vi "Inverter Test.vi"() -> ()   [LabVIEW 2016]
uses:
  <vilib>/TagLibrary/Create Tag (Int).vi
  <vilib>/TagLibrary/Write (Int).vi
  <vilib>/TagLibrary/Close Tag (Multiple).vi
  <vilib>/TagLibrary/TagLibrary.lvlib
  <resource>/objmgr/niTag.rc
panel:
  out "Iteration":i32
  in  "stop":bool
  out "Pass/Fail":bool
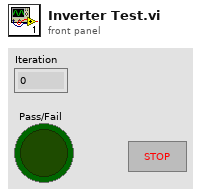
[diagram p1: front panel]
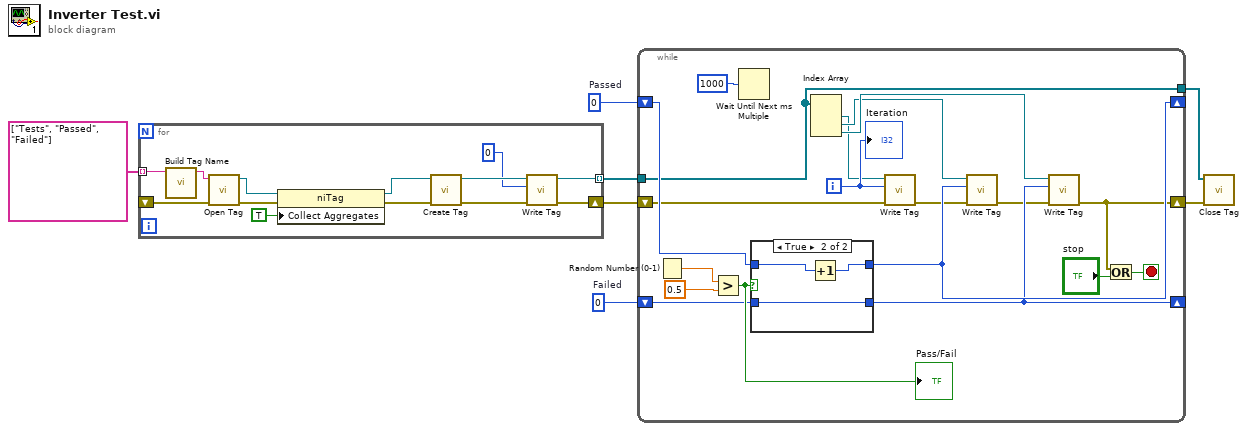
[diagram p0: block diagram]
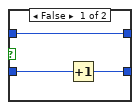
[diagram p2: hidden frame]
diagram:
  w5 = 0  # Failed
  w6 = 0  # Passed
  n1 = for {
    tunnel: string[] ["Tests", "Passed", "Failed"] -> [w19] mode=indexing
    tunnel: [w15] -> w4 mode=indexing
    shift-right: [w14] -> w2
    shift-left: _ -> [w13]
    n2 = call "Build Tag Name.vi"("Tag"=w19) -> ("System Tag"=w20:string)  [unwired: 10 in]
    n3 = call <vilib>:"Open Tag.vi"("error in (no error)"=w13, "tag path"=w20) -> ("error out"=w11:errorcluster, "tag reference out"=w12:refnum<k21>)  [unwired: 8 in]
    n4 = property class="niTag"(reference=w12, error in=w11, "Collect Aggregates"=TRUE) -> (reference out=w10:refnum<k21>, error out=w9:errorcluster)
    n5 = call-poly <vilib>:"Create Tag.vi"("error in (no error)"=w9, "tag reference in"=w10) -> ("error out"=w17:errorcluster, "tag reference out"=w18:refnum<k21>)  [unwired: 8 in]
    n6 = call-poly <vilib>:"Write Tag.vi"("error in (no error)"=w17, "int"=0, "tag reference in"=w18) -> ("error out"=w14:errorcluster, "tag reference out"=w15:refnum<k21>)  [unwired: 7 in]
  }
  n7 = while {
    tunnel: w4 -> [w27]
    shift-right: [w28] -> _
    shift-left: w5 -> [w33]
    shift-right: [w29] -> _
    shift-left: w6 -> [w34]
    tunnel: [w27] -> w3
    shift-right: [w21] -> w1
    shift-left: w2 -> [w26]
    i -> [w36]
    stop <- w23 stop-if-true
    n8 = Random Number (0-1)() -> (number: 0 to 1=w38:dbl)
    n9 = Greater?(x=w38, y=0.5) -> (0:w35:bool)
    "Pass/Fail" <- w35
    n10 = Wait Until Next ms Multiple(millisecond multiple=u32 1000) -> ()  [unwired: 1 out]
    n11 = case shown="True" w35 {
      tunnel: w34 -> [w40 w45]
      tunnel: [w40 w44] -> w29
      tunnel: w33 -> [w42 w43]
      tunnel: [w41 w43] -> w28
      frame False {
        n12 = Increment(x=w42) -> (x+1=w41:i32)
      }
      frame True {
        n13 = Increment(x=w45) -> (x+1=w44:i32)
      }
    }
    n14 = Index Array(array=w27) -> (element #1=w30:refnum<k21>, element #2=w31:refnum<k21>, element #3=w32:refnum<k21>)  [unwired: 3 in]
    n15 = call-poly <vilib>:"Write Tag.vi"("error in (no error)"=w26, "int"=w36, "tag reference in"=w30) -> ("error out"=w25:errorcluster)  [unwired: 7 in, 1 out]
    n16 = call-poly <vilib>:"Write Tag.vi"("error in (no error)"=w25, "int"=w29, "tag reference in"=w31) -> ("error out"=w24:errorcluster)  [unwired: 7 in, 1 out]
    n17 = call-poly <vilib>:"Write Tag.vi"("error in (no error)"=w24, "int"=w28, "tag reference in"=w32) -> ("error out"=w21:errorcluster)  [unwired: 7 in, 1 out]
    n18 = Or(x=w21, y="stop") -> (x .or. y?=w23:bool)
    "Iteration" <- w36
  }
  n19 = call-poly <vilib>:"Close Tag.vi"("error in (no error)"=w1, "tag references in"=w3) -> ()  [unwired: 9 in, 1 out]
